vi "5.PID-RT.vi"() -> ()   [LabVIEW 2014]
doc: "This example demonstrates how to simulate a general PID controller with alarms."
uses:
  vi.lib/Q-WaveSystems/QwaveSys Raspberry Pi for LabVIEW Home-Education/STM/_SubVIs/stm_MetaDataElement.ctl
  vi.lib/Q-WaveSystems/QwaveSys Raspberry Pi for LabVIEW Home-Education/CVT/_SubVIs/TypeDefs/cvt_Tag Configuration.ctl
  vi.lib/Q-WaveSystems/QwaveSys Raspberry Pi for LabVIEW Home-Education/CVT/_SubVIs/TypeDefs/cvt_Data Types.ctl
  <vilib>/Platform/TimedLoop/XDataNode/timing_clust.ctl
  <vilib>/Platform/TimedLoop/XDataNode/nitl_modes.ctl
  <vilib>/Platform/TimedLoop/XDataNode/wakeup.ctl
  vi.lib/Q-WaveSystems/QwaveSys Raspberry Pi for LabVIEW Home-Education/STM/TCP/STM Write Meta Data (TCP Ref).vi
  vi.lib/Q-WaveSystems/QwaveSys Raspberry Pi for LabVIEW Home-Education/STM/TCP/STM Write Message (TCP).vi
  vi.lib/Q-WaveSystems/QwaveSys Raspberry Pi for LabVIEW Home-Education/STM/TCP/STM Get Connection Reference (TCP).vi
  <vilib>/addons/control/pid/pid.llb/PID (DBL).vi
  <vilib>/platform/TimedLoop/XDataNode/XDataNode.xnode
  <vilib>/addons/control/pid/NI_PID_pid.lvlib
  <vilib>/Platform/TimedLoop/XDataNode/XDNodeRunTimeDep.lvlib
  vi.lib/Q-WaveSystems/QwaveSys Raspberry Pi for LabVIEW Home-Education/QwaveSys Raspberry Pi Library.lvlib
panel:
  in  "stop":bool
  in  "MIN":dbl(slide)=25.510204081632654 scale=0.0..100.0
  in  "MAX":dbl(slide)=87.75510204081633 scale=0.0..100.0
  out "Output (MV)":dbl(graph)
  out "Low Limit":bool
  out "High Limit":bool
  in  "SP:":dbl(slide)=54.966887417218544 min=0.0 max=0.0 scale=0.0..100.0
  out "MV:":dbl(slide)=100.0 scale=-100.0..100.0
  out "PV:":dbl(slide)=33.01408837398299 scale=0.0..100.0
  in  "PID gains":T1={"proportional gain (Kc)"=20.0, "integral time (Ti, min)"=0.008, "derivative time (Td, min)"=0.001} {"derivative time (Td, min)" format="%.3f"; "integral time (Ti, min)" format="%.3f"; "proportional gain (Kc)" format="%.3f"}
  out "Monitor Chart":cluster{"initial PV":dbl, "SP:":dbl, dbl, dbl}(graph)
  # "Overview: This example demonstrates how to simulate a general PID controller with alarms.\nInstructions:\n1. Run the VI and observe the Process Variable (PV) following the Setpoint (SP) value.\n2. Move the setpoint above or below the High Limit (HL) or Low Limit (LL). Verify the controls flashing when limits are reached.\n3. Change the Alarm limits to a value above or below if you are changing HL or LL, respectively and verify that the controller stop flashing.\n3. Click Stop to stop the VI."
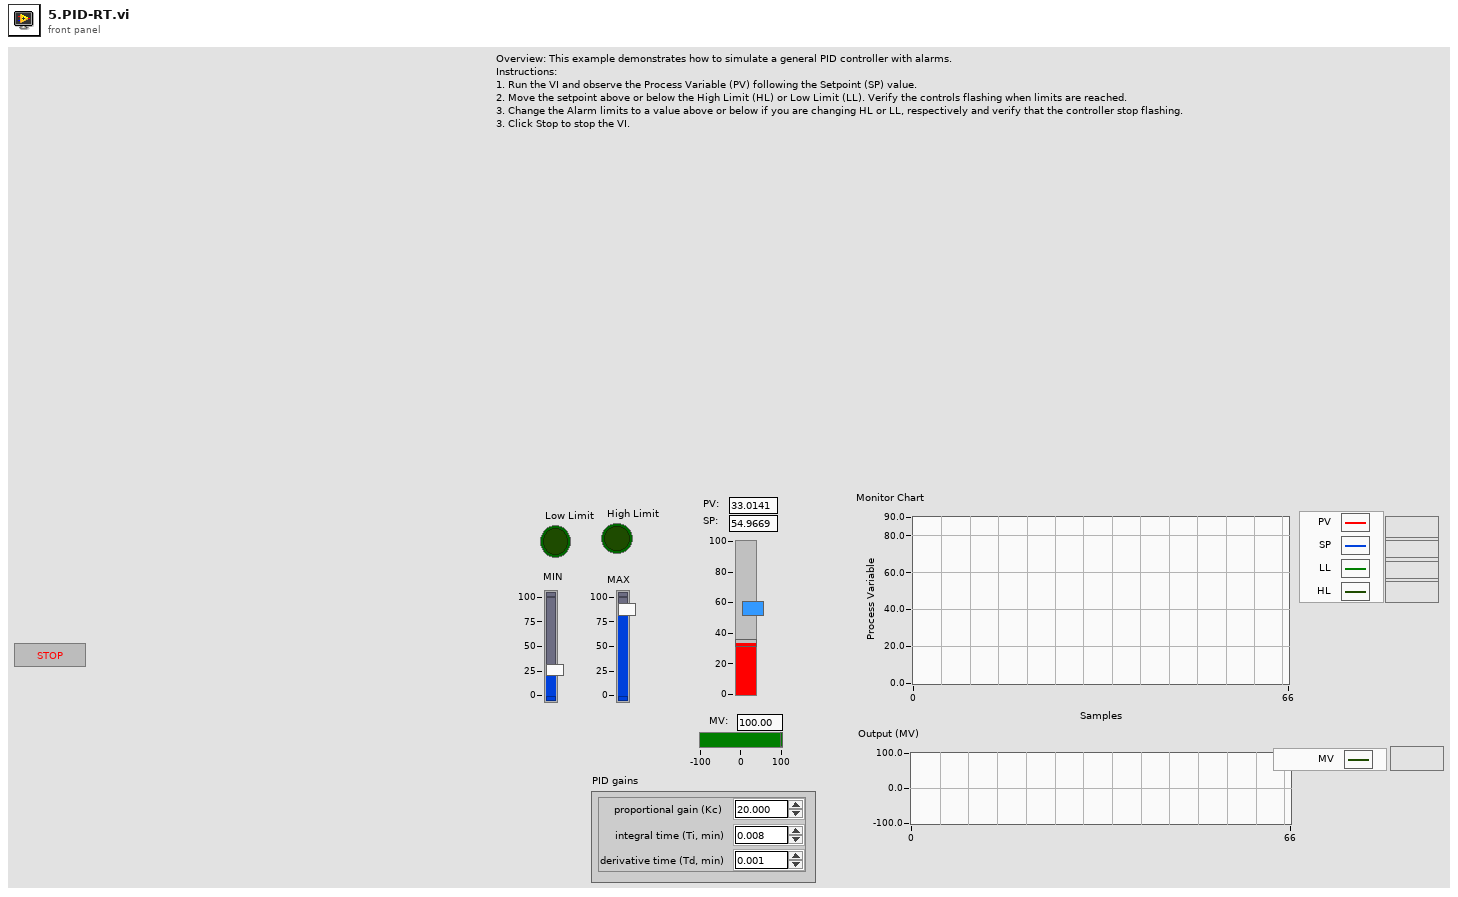
[diagram p1: front panel]
types:
  T1 = cluster{"proportional gain (Kc)":dbl, "integral time (Ti, min)":dbl, "derivative time (Td, min)":dbl}
  T2 = typedef "QwaveSys Raspberry Pi Library.lvlib/cvt_Tag Configuration.ctl" = cluster{"Name":string, "Data Type":T3, "Array":bool, "Size":u32, "Default":string, "Enum":string[], "Description":string}
  T3 = typedef "QwaveSys Raspberry Pi Library.lvlib/cvt_Data Types.ctl" = enum16{"Bool", "U8", "I32", "Double", "String", "Enum"}
  T4 = typedef "QwaveSys Raspberry Pi Library.lvlib/stm_MetaDataElement.ctl" = string
  T5 = typedef "XDNodeRunTimeDep.lvlib/timing_clust.ctl" = cluster{"Expected End [f-1]":u64, "Actual End [f-1]":u64, "Finished Late? [f-1]":bool, "Expected End [i-1]":u64, "Actual End [i-1]":u64, "Finished Late? [i-1]":bool, "Expected Start [i]":u64, "Actual Start [i]":u64, "Expected Start [f]":u64, "Actual Start [f]":u64, "Source Name":string, "Structure Name":string, "Period":i64, "Deadline":i64, "Offset":i64, "Start":i64, "Priority":i32, "Timeout":i32, "Mode":T6, "Wakeup Reason":T7, "Error":errorcluster, "Source Type":string, "Secondary Source Type":string, "Global End Time":u64, "Global Start Time":u64, "Frame Duration":u64, "Iteration Duration":u64, "Assigned CPU":i32, "I/O Scan Engine Mode":u32}
  T6 = typedef "XDNodeRunTimeDep.lvlib/nitl_modes.ctl" = enum32{"No Change", "Process missed periods, maintain original phase", "Discard missed periods, maintain original phase", "Process missed periods, ignore original phase", "Discard missed periods, ignore original phase"}
  T7 = typedef "XDNodeRunTimeDep.lvlib/wakeup.ctl" = enum32{"Normal", "Aborted", "Asynchronous wakeup", "Timing source error", "Timed loop error", "Timeout"}
  T8 = typedef "QwaveSys Raspberry Pi Library.lvlib/stm_TCP Connection Info.ctl" = cluster{"connection ID":refnum<k5>, "Meta data":T4[]}
  T9 = cluster{"static gain":dbl, "lag (min)":dbl, "dead cycles":dbl, "load %":dbl, "deadband":dbl, "noise level %":dbl, "initial PV":dbl, "initial PV 2":dbl}
  T10 = cluster{"Plant Output":dbl, "SP:":dbl, "MIN":dbl, "MAX":dbl}
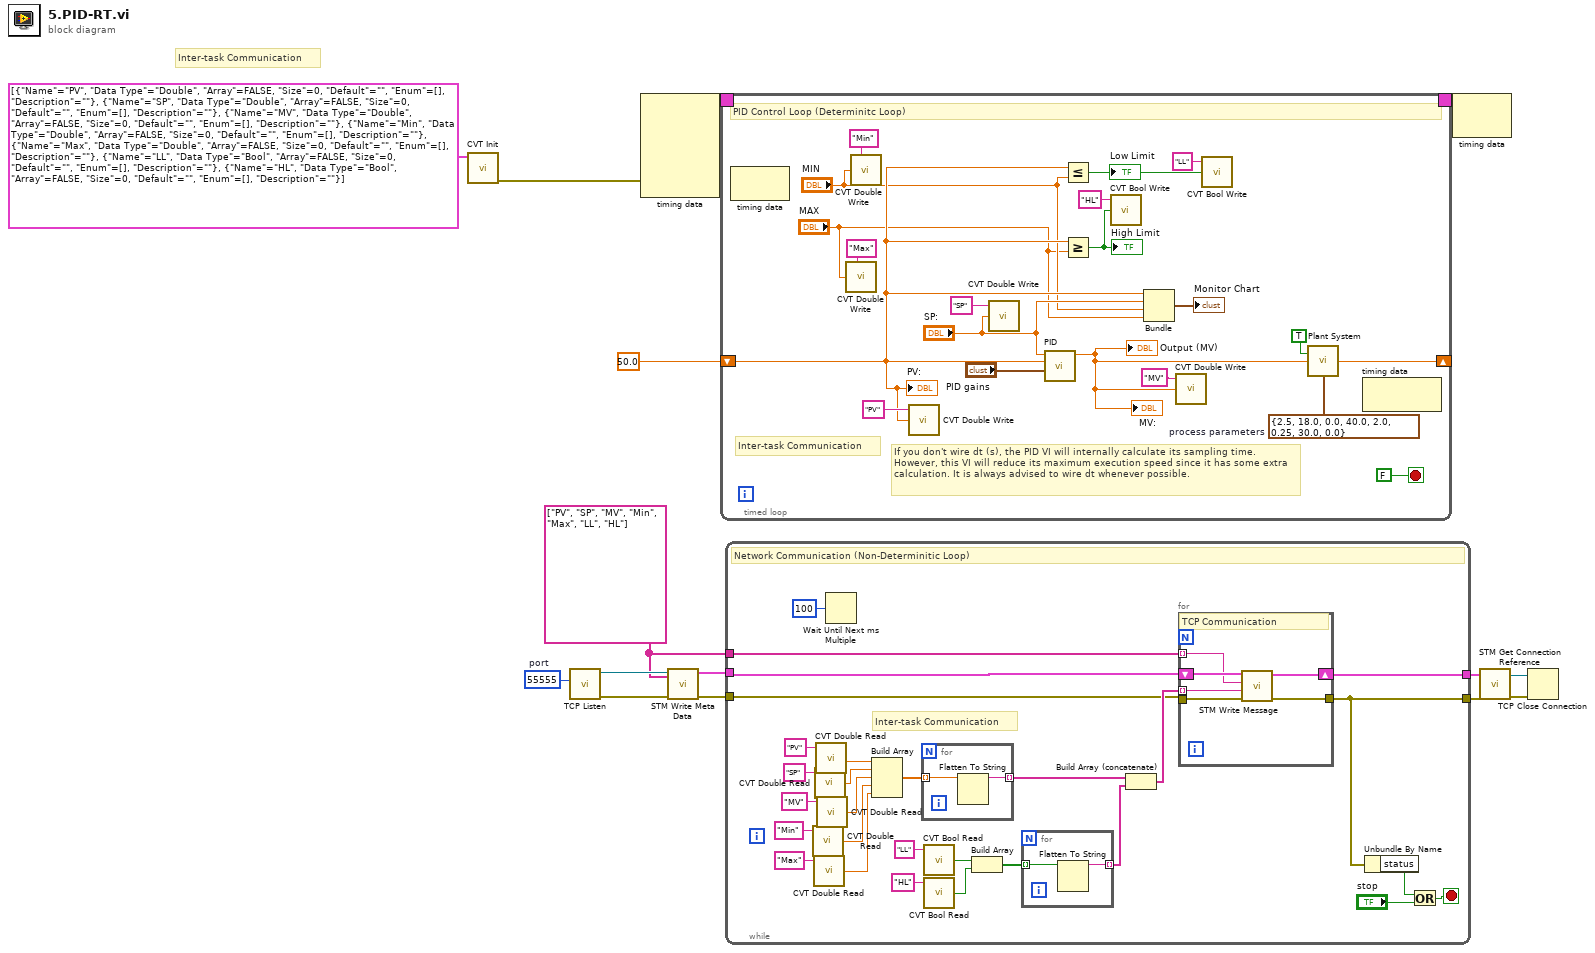
[diagram p0: block diagram]
diagram:
  w1 = T4[] ["PV", "SP", "MV", "Min", "Max", "LL", "HL"] ("Meta data")
  w12 = u16 55555  # port
  # "Inter-task Communication"
  n1 = call "CVT Init.vi"("Tag List"=T2[] [{"Name"="PV", "Data Type"=enum."Double", "Array"=FALSE, "Size"=0, "Default"="", "Enum"=[], "Description"=""}, {"Name"="SP", "Data Type"=enum."Double", "Array"=FALSE, "Size"=0, "Default"="", "Enum"=[], "Description"=""}, {"Name"="MV", "Data Type"=enum."Double", "Array"=FALSE, "Size"=0, "Default"="", "Enum"=[], "Description"=""}, {"Name"="Min", "Data Type"=enum."Double", "Array"=FALSE, "Size"=0, "Default"="", "Enum"=[], "Description"=""}, {"Name"="Max", "Data Type"=enum."Double", "Array"=FALSE, "Size"=0, "Default"="", "Enum"=[], "Description"=""}, {"Name"="LL", "Data Type"=enum."Bool", "Array"=FALSE, "Size"=0, "Default"="", "Enum"=[], "Description"=""}, {"Name"="HL", "Data Type"=enum."Bool", "Array"=FALSE, "Size"=0, "Default"="", "Enum"=[], "Description"=""}]) -> ("error out"=w5:errorcluster)  [unwired: 1 in, 9 out]
  n2 = call <vilib>:"TCP Listen.vi"("port"=w12) -> ("error out"=w10:errorcluster, "connection ID"=w11:refnum<k5>)  [unwired: 3 in, 6 out]
  n3 = node-c288(w5) -> (w14:T5)  [unwired: 4 in]
  n4 = call-poly "STM Write Meta Data.vi"("Meta data"=w1, "error in"=w10, "connection ID"=w11) -> ("error out"=w8:errorcluster, "Connection Info Out"=w9:T8)  [unwired: 1 in, 6 out]
  n5 = timed-loop {
    shift-left: 50.0 ("Plant Output") -> [w28]
    shift-right: [w34] -> _
    timing: w14 -> [_]
    timing-out: [_] -> w13
    stop <- FALSE stop-if-true
    w32 = T9 {"static gain"=2.5, "lag (min)"=18.0, "dead cycles"=0.0, "load %"=40.0, "deadband"=2.0, "noise level %"=0.25, "initial PV"=30.0, "initial PV 2"=0.0}  # process parameters
    # "Inter-task Communication"
    # "If you don't wire dt (s), the PID VI will internally calculate its sampling time. However, this VI will reduce its maximum execution speed since it has some extra calculation. It is always advised to wire dt whenever possible."
    # "PID Control Loop (Determinitc Loop)"
    n6 = node-c288() -> ()  [unwired: 1 in, 1 out]
    n7 = call "CVT Double Write.vi"("Value"="MAX", "Tag Name"="Max") -> ()  [unwired: 3 in, 1 out]
    n8 = call "CVT Double Write.vi"("Value"="MIN", "Tag Name"="Min") -> ()  [unwired: 3 in, 1 out]
    n9 = call "CVT Double Write.vi"("Value"=w28, "Tag Name"="PV") -> ()  [unwired: 3 in, 1 out]
    n10 = call "CVT Double Write.vi"("Value"="SP:", "Tag Name"="SP") -> ()  [unwired: 3 in, 1 out]
    n11 = call-poly <vilib>:"PID.vi"("PID gains"="PID gains", "process variable"=w28, "setpoint"="SP:") -> ("output"=w24:dbl)  [unwired: 7 in, 1 out]
    "MV:" <- w24
    "Output (MV)" <- w24
    n12 = Less Or Equal?(x=w28, y="MIN") -> (x <= y?=w17:bool)
    "Low Limit" <- w17
    n13 = Greater Or Equal?(x=w28, y="MAX") -> (x >= y?=w16:bool)
    "High Limit" <- w16
    n14 = call "CVT Bool Write.vi"("Value"=w16, "Tag Name"="HL") -> ()  [unwired: 3 in, 1 out]
    n15 = Bundle("Plant Output"=w28, "SP:"="SP:", "MIN"="MIN", "MAX"="MAX") -> (→"Monitor Chart":T10)  [unwired: 1 in]
    n16 = call "CVT Double Write.vi"("Value"=w24, "Tag Name"="MV") -> ()  [unwired: 3 in, 1 out]
    n17 = call "CVT Bool Write.vi"("Value"=w17, "Tag Name"="LL") -> ()  [unwired: 3 in, 1 out]
    n18 = call "Plant System.vi"("Integrator ?"=TRUE, "Plant Input"=w24, "process parameters"=w32) -> ("Plant Output"=w34:dbl)  [unwired: 12 in]
    n19 = node-c288() -> ()  [unwired: 1 in, 1 out]
    "PV:" <- w28
  }
  n20 = while {
    tunnel: w9 -> [w45]
    tunnel: w8 -> [w44]
    tunnel: [w43] -> w3
    tunnel: [w39] -> w2
    tunnel: w1 -> [w42]
    stop <- w38 stop-if-true
    # "Inter-task Communication"
    # "Network Communication (Non-Determinitic Loop)"
    n21 = call "CVT Double Read.vi"("Tag Name"="Min") -> ("Value"=w56:dbl)  [unwired: 3 in, 1 out]
    n22 = call "CVT Double Read.vi"("Tag Name"="Max") -> ("Value"=w55:dbl)  [unwired: 3 in, 1 out]
    n23 = call "CVT Double Read.vi"("Tag Name"="SP") -> ("Value"=w58:dbl)  [unwired: 3 in, 1 out]
    n24 = call "CVT Double Read.vi"("Tag Name"="PV") -> ("Value"=w63:dbl)  [unwired: 3 in, 1 out]
    n25 = call "CVT Double Read.vi"("Tag Name"="MV") -> ("Value"=w57:dbl)  [unwired: 3 in, 1 out]
    n26 = Wait Until Next ms Multiple(millisecond multiple=u32 100) -> ()  [unwired: 1 out]
    n27 = Build Array(w63, w58, w57, w56, w55) -> (w52:dbl[])
    n28 = for {
      tunnel: w52 -> [w69] mode=indexing
      tunnel: [w68] -> w51 mode=indexing
      n29 = Flatten To String(anything=w69) -> (data string=w68:string)  [unwired: 1 in, 4 out]
    }
    n30 = call "CVT Bool Read.vi"("Tag Name"="LL") -> ("Value"=w49:bool)  [unwired: 3 in, 1 out]
    n31 = call "CVT Bool Read.vi"("Tag Name"="HL") -> ("Value"=w48:bool)  [unwired: 3 in, 1 out]
    n32 = Build Array(w49, w48) -> (w50:bool[])
    n33 = for {
      tunnel: w50 -> [w67] mode=indexing
      tunnel: [w66] -> w47 mode=indexing
      n34 = Flatten To String(anything=w67) -> (data string=w66:string)  [unwired: 1 in, 4 out]
    }
    n35 = Build Array (concatenate)(w51, w47) -> (w46:string[])
    n36 = for {
      tunnel: [w74] -> w39
      tunnel: w44 -> [w73]
      tunnel: w46 -> [w71] mode=indexing
      shift-right: [w75] -> w43
      shift-left: w45 -> [w72]
      tunnel: w42 -> [w70] mode=indexing
      # "TCP Communication"
      n37 = call-poly "STM Write Message.vi"("error in (no error)"=w73, "Data"=w71, "Name"=w70, "Connection Info"=w72) -> ("error out"=w74:errorcluster, "Connection Info Out"=w75:T8)  [unwired: 1 in, 5 out]
    }
    n38 = Unbundle By Name(w39) -> ("status"=w40:bool)
    n39 = Or(x=w40, y="stop") -> (x .or. y?=w38:bool)
  }
  n40 = node-c288(w13) -> ()  [unwired: 1 out]
  n41 = call-poly "STM Get Connection Reference.vi"("error in"=w2, "Connection Info"=w3) -> ("error out"=w6:errorcluster, "connection ID out"=w7:refnum<k5>)  [unwired: 8 out]
  n42 = TCP Close Connection(connection ID=w7, error in (no error)=w6) -> ()  [unwired: 3 out]
